vi "hw3-1 topVI.vi"() -> ()   [LabVIEW 2014]
panel:
  out "input":dbl[](array[numeric])
  out "XY Graph":cluster{i32[], dbl[]}(graph)
  out "temp":dbl[](array[numeric])
  out "sorted":dbl[](array[numeric])
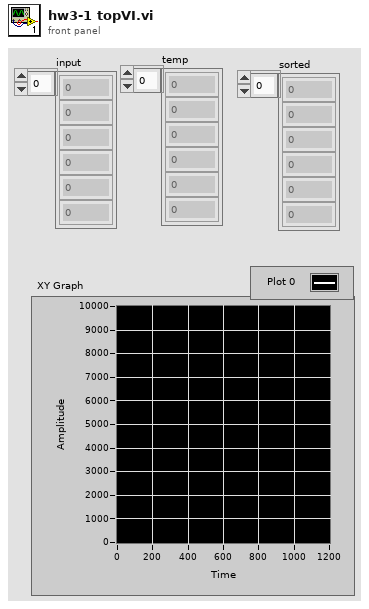
[diagram p1: front panel]
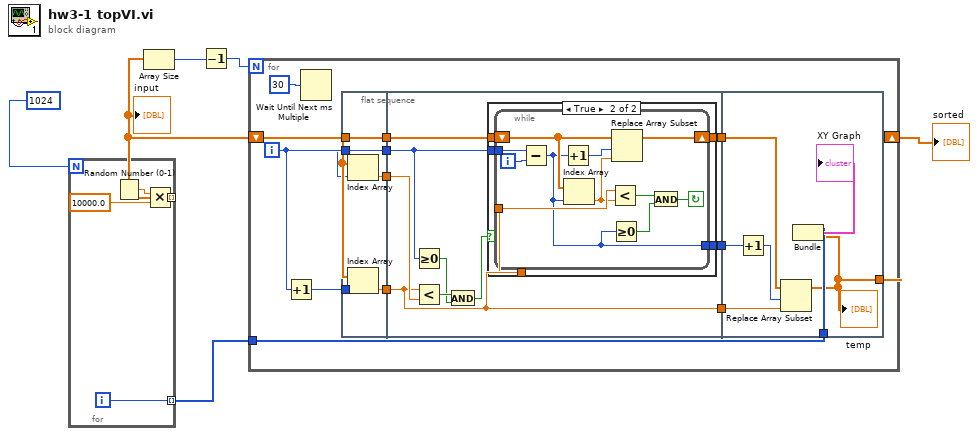
[diagram p0: block diagram]
diagram:
  n1 = for {
    N: 1024 -> [_]
    tunnel: [w8] -> w2 mode=indexing
    tunnel: [w7] -> w1 mode=indexing
    i -> [w7]
    n2 = Random Number (0-1)() -> (number: 0 to 1=w10:dbl)
    n3 = Multiply(x=w10, y=10000.0) -> (x*y=w8:dbl)
  }
  "input" <- w2
  n4 = Array Size(array=w2) -> (size(s)=w5:i32)
  n5 = Decrement(x=w5) -> (x-1=w6:i32)
  n6 = for {
    N: w6 -> [_]
    shift-right: [w13] -> w4
    shift-left: w2 -> [w21]
    tunnel: w1 -> [w12]
    i -> [w22]
    n7 = Increment(x=w22) -> (x+1=w23:i32)
    n8 = Wait Until Next ms Multiple(millisecond multiple=u32 30) -> ()  [unwired: 1 out]
    n9 = flat-sequence {
      tunnel: w23 -> [w25]
      tunnel: w22 -> [w24]
      tunnel: w21 -> [w26]
      tunnel: [w28] -> w20
      tunnel: [w27] -> w19
      tunnel: [w26] -> w18
      tunnel: [w24] -> w17
      tunnel: w20 -> [w33]
      tunnel: w19 -> [w29]
      tunnel: w18 -> [w34]
      tunnel: w17 -> [w32]
      tunnel: [w31] -> w16
      tunnel: [w30] -> w15
      tunnel: [w29] -> w14
      tunnel: w16 -> [w60]
      tunnel: w15 -> [w61]
      tunnel: w14 -> [w59]
      tunnel: [w56] -> w13
      tunnel: w12 -> [w57]
      frame #0 {
        n10 = Index Array(array=w26, index=w24) -> (element=w28:dbl)
        n11 = Index Array(array=w26, index=w25) -> (element=w27:dbl)
      }
      frame #1 {
        n12 = Greater Or Equal To 0?(x=w32) -> (x >= 0?=w36:bool)
        n13 = Less?(x=w29, y=w33) -> (x < y?=w37:bool)
        n14 = And(x=w37, y=w36) -> (x .and. y?=w35:bool)
        n15 = case shown="True" w35 {
          tunnel: w32 -> [w39 w44]
          tunnel: w34 -> [w38 w43]
          tunnel: w29 -> [_ w42]
          tunnel: [w39 w41] -> w31
          tunnel: [w38 w40] -> w30
          frame False {
          }
          frame True {
            n16 = while {
              shift-right: [w51] -> w40
              shift-left: w43 -> [w52]
              tunnel: w44 -> [w55]
              tunnel: w42 -> [w50]
              tunnel: [w45] -> w41
              i -> [w54]
              stop <- w46 continue-if-true
              n17 = Subtract(x=w55, y=w54) -> (x-y=w45:i32)
              n18 = Increment(x=w45) -> (x+1=w53:i32)
              n19 = Index Array(array=w52, index=w45) -> (element=w49:dbl)
              n20 = Less?(x=w50, y=w49) -> (x < y?=w48:bool)
              n21 = Greater Or Equal To 0?(x=w45) -> (x >= 0?=w47:bool)
              n22 = Replace Array Subset(array=w52, new element=w49, index=w53) -> (w51:dbl[])
              n23 = And(x=w48, y=w47) -> (x .and. y?=w46:bool)
            }
          }
        }
      }
      frame #2 {
        n24 = Increment(x=w60) -> (x+1=w62:i32)
        n25 = Replace Array Subset(array=w61, new element=w59, index=w62) -> (w56:dbl[])
        "temp" <- w56
        n26 = Bundle(w57, w56) -> (→"XY Graph":cluster{i32[], dbl[]})  [unwired: 1 in]
      }
    }
  }
  "sorted" <- w4
